vi "LatticeRamp_Generate_v4.vi"(5 "Input ramp":T4={"lattice ramp"=[{"dt"="0.010", "formula"="0.0"}, {"dt"="0.010", "formula"="f"}, {"dt"="0.010", "formula"="sin(2*pi*100*t)+1"}, {"dt"="0.010", "formula"="1-f"}], "Output"=[{"Time Values"=[0.0, 7.4775e-05, 0.004952823780487805, 0.009830872560975609, 0.014708921341463415, 0.01958697012195122, 0.024465018902439024, 0.02934306768292683, 0.034221116463414636, 0.03909916524390244, 0.04397721402439025, 0.04885526280487805, 0.05373331158536586, 0.05861136036585366, 0.06348940914634146, 0.06836745792682927, 0.07324550670731708, 0.07812355548780488, 0.08300160426829269, 0.0878796530487805, 0.09275770182926829, 0.0976357506097561, 0.10251379939024391, 0.10739184817073172, 0.11226989695121951, 0.11714794573170732, 0.12202599451219513, 0.12690404329268293, 0.13178209207317074, 0.13666014085365855, 0.14153818963414636, 0.14641623841463416, 0.15129428719512195, 0.15617233597560976, 0.16105038475609756, 0.16592843353658537, 0.17080648231707318, 0.175684531097561, 0.1805625798780488, 0.18544062865853658, 0.1903186774390244, 0.1951967262195122, 0.200074775, 0.20014955, 0.20504955, 0.20994955, 0.210024325, 0.710524325, 1.211024325, 1.2110991, 1.2111991, 1.2112991], [-2.42, -2.42, -2.274644675841946, -2.209161629253642, -2.1550360243297555, -2.1059224619056875, -2.059369043262097, -2.0141023350157363, -1.9693429960844966, -1.9245576980378343, -1.8793492014535609, -1.8334007369631589, -1.7864449866349144, -1.7382453890245562, -1.6885840896654052, -1.6372536703029252, -1.5840511006332372, -1.5287730108087192, -1.4712117270212386, -1.4111516989449542, -1.3483660486208333, -1.2826130206804396, -1.2136321308648308, -1.14113980114949, -1.064824236902151, -0.9843392409185628, -0.899296562073762, -0.809256226432418, -0.7137140678937928, -0.6120853153944805, -0.503682519181236, -0.38768515498282585, -0.26309663961745094, -0.1286816451362946, 0.017128703533097003, 0.17638664147159178, 0.35187774884695067, 0.547568099398879, 0.7694813778413232, 1.027657386702481, 1.3414861643128648, 1.7605557393789637, 2.8, 2.8, 2.8, 2.8, 2.8, 2.8, 2.8, -2.42, -2.42, -2.42]}, {"Time Values"=[0.0, 7.4775e-05, 0.004952823780487805, 0.009830872560975609, 0.014708921341463415, 0.01958697012195122, 0.024465018902439024, 0.02934306768292683, 0.034221116463414636, 0.03909916524390244, 0.04397721402439025, 0.04885526280487805, 0.05373331158536586, 0.05861136036585366, 0.06348940914634146, 0.06836745792682927, 0.07324550670731708, 0.07812355548780488, 0.08300160426829269, 0.0878796530487805, 0.09275770182926829, 0.0976357506097561, 0.10251379939024391, 0.10739184817073172, 0.11226989695121951, 0.11714794573170732, 0.12202599451219513, 0.12690404329268293, 0.13178209207317074, 0.13666014085365855, 0.14153818963414636, 0.14641623841463416, 0.15129428719512195, 0.15617233597560976, 0.16105038475609756, 0.16592843353658537, 0.17080648231707318, 0.175684531097561, 0.1805625798780488, 0.18544062865853658, 0.1903186774390244, 0.1951967262195122, 0.200074775, 0.20014955, 0.20504955, 0.20994955, 0.210024325, 0.710524325, 1.211024325, 1.2110991, 1.2111991, 1.2112991], [0.0, -0.0, 0.001911981360536598, 0.004019900016154734, 0.006343835359047381, 0.008905924490689818, 0.011730573093137419, 0.01484468791013227, 0.018277933052562964, 0.022063012569765436, 0.026235981978353178, 0.030836591716105637, 0.03590866579255229, 0.04150051924316252, 0.04766541836368316, 0.05446208810867599, 0.06195527148757928, 0.0702163462869304, 0.07932400499345772, 0.08936500439478239, 0.10043499199819844, 0.11263941713974554, 0.12609453546252153, 0.1409285163325908, 0.15728266374139496, 0.17531276232461152, 0.19519056131922613, 0.21710541059454333, 0.24126606434146913, 0.2679026696014608, 0.2972689585772668, 0.3296446656087423, 0.36533819183711563, 0.40468954294049037, 0.44807356792455355, 0.4959035298202305, 0.5486350423016632, 0.6067704097235386, 0.6708634119196445, 0.7415245793411871, 0.8194270087842359, 0.905312775105144, 1.0, 1.0, 1.0, 1.0, 1.0, 1.0, 1.0, 0.0, 0.0, 0.0]}], "SRS Selection"=enum."1550 Vertical"}, 6 "Current Variable settings":T1[](array[typedef])=[{"Procedure variable"="delay", "Value"=2.3}, {"Procedure variable"="z", "Value"=0.0}], 7 "error in (no error)":errorcluster) -> (0 "Output ramp":T4={"lattice ramp"=[{"dt"="0.010", "formula"="0.0"}, {"dt"="0.010", "formula"="f"}, {"dt"="0.010", "formula"="sin(2*pi*100*t)+1"}, {"dt"="0.010", "formula"="1-f"}], "Output"=[{"Time Values"=[0.0, 2.475e-06, 0.000771248076923077, 0.001540021153846154, 0.0023087942307692313, 0.003077567307692308, 0.003846340384615385, 0.0046151134615384625, 0.005383886538461539, 0.006152659615384616, 0.006921432692307693, 0.00769020576923077, 0.008458978846153847, 0.009227751923076925, 0.009996525000000001, 0.009999000000000001, 0.010768344230769231, 0.011537688461538463, 0.012307032692307693, 0.013076376923076925, 0.013845721153846155, 0.014615065384615385, 0.015384409615384616, 0.016153753846153848, 0.016923098076923077, 0.01769244230769231, 0.01846178653846154, 0.01923113076923077, 0.020000475, 0.02000295, 0.02018466, 0.020366369999999998, 0.02054808, 0.020729789999999998, 0.0209115, 0.021093209999999998, 0.02127492, 0.021456629999999997, 0.02163834, 0.02182005, 0.02200176, 0.022183469999999997, 0.02236518, 0.02254689, 0.022728599999999998, 0.02291031, 0.023092019999999998, 0.02327373, 0.023455439999999998, 0.02363715, 0.023818859999999997, 0.02400057, 0.02418228, 0.02436399, 0.0245457, 0.02472741, 0.02490912, 0.025090829999999998, 0.02527254, 0.025454249999999998, 0.02563596, 0.02581767, 0.02599938, 0.026181089999999997, 0.0263628, 0.02654451, 0.02672622, 0.02690793, 0.027089639999999998, 0.02727135, 0.02745306, 0.02763477, 0.027816479999999998, 0.02799819, 0.0281799, 0.02836161, 0.028543319999999997, 0.02872503, 0.02890674, 0.029088450000000002, 0.02927016, 0.029451869999999998, 0.02963358, 0.02981529, 0.029997, 0.029999474999999998, 0.03076881923076923, 0.03153816346153846, 0.03230750769230769, 0.03307685192307692, 0.03384619615384615, 0.03461554038461538, 0.03538488461538461, 0.036154228846153845, 0.03692357307692307, 0.03769291730769231, 0.03846226153846154, 0.039231605769230765, 0.04000094999999999], [0.0, 0.0, 0.0, 0.0, 0.0, 0.0, 0.0, 0.0, 0.0, 0.0, 0.0, 0.0, 0.0, 0.0, 0.0, 0.0, 0.07692307692307693, 0.15384615384615385, 0.23076923076923078, 0.3076923076923077, 0.38461538461538464, 0.46153846153846156, 0.5384615384615384, 0.6153846153846154, 0.6923076923076923, 0.7692307692307693, 0.8461538461538461, 0.9230769230769231, 1.0, 1.0, 1.1139238800498696, 1.226364353008397, 1.335857327283306, 1.4409770907726172, 1.5403548751151055, 1.6326966784741854, 1.716800114784089, 1.7915700700636759, 1.8560329619364289, 1.9093494166828902, 1.950825198757172, 1.9799202504538926, 1.9962557240197008, 1.9996189146440044, 1.9899660300962418, 1.9674227609461497, 1.9322826439421659, 1.8850032398584795, 1.8262001755791255, 1.7566391279973623, 1.6772258541082894, 1.588994397113228, 1.4930936221046294, 1.3907722566508556, 1.2833626310679325, 1.1722633300968168, 1.0589209818793124, 0.9448114213590806, 0.8314204733797951, 0.7202246057044277, 0.6126717038734424, 0.5101622182331631, 0.41403092861958235, 0.3255295641403312, 0.245810504363279, 0.17591177413920145, 0.11674352744147698, 0.06907619621725625, 0.03353045856433845, 0.010569156858512452, 0.0004912710657166697, 0.003428025712751026, 0.019341181207819358, 0.048023531759680216, 0.0891016034119837, 0.14204051706158627, 0.20615095313930343, 0.2805981272657321, 0.36441266000978945, 0.4565031992144406, 0.5556706305338442, 0.6606236911459755, 0.7699957833339905, 0.8823627690060711, 0.9962615134506403, 1.0, 0.9230769230769231, 0.8461538461538461, 0.7692307692307692, 0.6923076923076923, 0.6153846153846154, 0.5384615384615384, 0.46153846153846156, 0.3846153846153846, 0.3076923076923077, 0.23076923076923073, 0.15384615384615385, 0.07692307692307687, 0.0]}, {"Time Values"=[0.0, 2.475e-06, 0.000771248076923077, 0.001540021153846154, 0.0023087942307692313, 0.003077567307692308, 0.003846340384615385, 0.0046151134615384625, 0.005383886538461539, 0.006152659615384616, 0.006921432692307693, 0.00769020576923077, 0.008458978846153847, 0.009227751923076925, 0.009996525000000001, 0.009999000000000001, 0.010768344230769231, 0.011537688461538463, 0.012307032692307693, 0.013076376923076925, 0.013845721153846155, 0.014615065384615385, 0.015384409615384616, 0.016153753846153848, 0.016923098076923077, 0.01769244230769231, 0.01846178653846154, 0.01923113076923077, 0.020000475, 0.02000295, 0.02018466, 0.020366369999999998, 0.02054808, 0.020729789999999998, 0.0209115, 0.021093209999999998, 0.02127492, 0.021456629999999997, 0.02163834, 0.02182005, 0.02200176, 0.022183469999999997, 0.02236518, 0.02254689, 0.022728599999999998, 0.02291031, 0.023092019999999998, 0.02327373, 0.023455439999999998, 0.02363715, 0.023818859999999997, 0.02400057, 0.02418228, 0.02436399, 0.0245457, 0.02472741, 0.02490912, 0.025090829999999998, 0.02527254, 0.025454249999999998, 0.02563596, 0.02581767, 0.02599938, 0.026181089999999997, 0.0263628, 0.02654451, 0.02672622, 0.02690793, 0.027089639999999998, 0.02727135, 0.02745306, 0.02763477, 0.027816479999999998, 0.02799819, 0.0281799, 0.02836161, 0.028543319999999997, 0.02872503, 0.02890674, 0.029088450000000002, 0.02927016, 0.029451869999999998, 0.02963358, 0.02981529, 0.029997, 0.029999474999999998, 0.03076881923076923, 0.03153816346153846, 0.03230750769230769, 0.03307685192307692, 0.03384619615384615, 0.03461554038461538, 0.03538488461538461, 0.036154228846153845, 0.03692357307692307, 0.03769291730769231, 0.03846226153846154, 0.039231605769230765, 0.04000094999999999], [0.0, 0.0, 0.0, 0.0, 0.0, 0.0, 0.0, 0.0, 0.0, 0.0, 0.0, 0.0, 0.0, 0.0, 0.0, 0.0, 0.07692307692307693, 0.15384615384615385, 0.23076923076923078, 0.3076923076923077, 0.38461538461538464, 0.46153846153846156, 0.5384615384615384, 0.6153846153846154, 0.6923076923076923, 0.7692307692307693, 0.8461538461538461, 0.9230769230769231, 1.0, 1.0, 1.1139238800498696, 1.226364353008397, 1.335857327283306, 1.4409770907726172, 1.5403548751151055, 1.6326966784741854, 1.716800114784089, 1.7915700700636759, 1.8560329619364289, 1.9093494166828902, 1.950825198757172, 1.9799202504538926, 1.9962557240197008, 1.9996189146440044, 1.9899660300962418, 1.9674227609461497, 1.9322826439421659, 1.8850032398584795, 1.8262001755791255, 1.7566391279973623, 1.6772258541082894, 1.588994397113228, 1.4930936221046294, 1.3907722566508556, 1.2833626310679325, 1.1722633300968168, 1.0589209818793124, 0.9448114213590806, 0.8314204733797951, 0.7202246057044277, 0.6126717038734424, 0.5101622182331631, 0.41403092861958235, 0.3255295641403312, 0.245810504363279, 0.17591177413920145, 0.11674352744147698, 0.06907619621725625, 0.03353045856433845, 0.010569156858512452, 0.0004912710657166697, 0.003428025712751026, 0.019341181207819358, 0.048023531759680216, 0.0891016034119837, 0.14204051706158627, 0.20615095313930343, 0.2805981272657321, 0.36441266000978945, 0.4565031992144406, 0.5556706305338442, 0.6606236911459755, 0.7699957833339905, 0.8823627690060711, 0.9962615134506403, 1.0, 0.9230769230769231, 0.8461538461538461, 0.7692307692307692, 0.6923076923076923, 0.6153846153846154, 0.5384615384615384, 0.46153846153846156, 0.3846153846153846, 0.3076923076923077, 0.23076923076923073, 0.15384615384615385, 0.07692307692307687, 0.0]}], "SRS Selection"=enum."1550 Vertical"}, 1 "Output time":dbl[](array[numeric])=[0.0, 2.475e-06, 0.000771248076923077, 0.001540021153846154, 0.0023087942307692313, 0.003077567307692308, 0.003846340384615385, 0.0046151134615384625, 0.005383886538461539, 0.006152659615384616, 0.006921432692307693, 0.00769020576923077, 0.008458978846153847, 0.009227751923076925, 0.009996525000000001, 0.009999000000000001, 0.010768344230769231, 0.011537688461538463, 0.012307032692307693, 0.013076376923076925, 0.013845721153846155, 0.014615065384615385, 0.015384409615384616, 0.016153753846153848, 0.016923098076923077, 0.01769244230769231, 0.01846178653846154, 0.01923113076923077, 0.020000475, 0.02000295, 0.02018466, 0.020366369999999998, 0.02054808, 0.020729789999999998, 0.0209115, 0.021093209999999998, 0.02127492, 0.021456629999999997, 0.02163834, 0.02182005, 0.02200176, 0.022183469999999997, 0.02236518, 0.02254689, 0.022728599999999998, 0.02291031, 0.023092019999999998, 0.02327373, 0.023455439999999998, 0.02363715, 0.023818859999999997, 0.02400057, 0.02418228, 0.02436399, 0.0245457, 0.02472741, 0.02490912, 0.025090829999999998, 0.02527254, 0.025454249999999998, 0.02563596, 0.02581767, 0.02599938, 0.026181089999999997, 0.0263628, 0.02654451, 0.02672622, 0.02690793, 0.027089639999999998, 0.02727135, 0.02745306, 0.02763477, 0.027816479999999998, 0.02799819, 0.0281799, 0.02836161, 0.028543319999999997, 0.02872503, 0.02890674, 0.029088450000000002, 0.02927016, 0.029451869999999998, 0.02963358, 0.02981529, 0.029997, 0.029999474999999998, 0.03076881923076923, 0.03153816346153846, 0.03230750769230769, 0.03307685192307692, 0.03384619615384615, 0.03461554038461538, 0.03538488461538461, 0.036154228846153845, 0.03692357307692307, 0.03769291730769231, 0.03846226153846154, 0.039231605769230765, 0.04000094999999999] format="%#_6p", 2 "Output calculated":dbl[](array[numeric])=[0.0, 0.0, 0.0, 0.0, 0.0, 0.0, 0.0, 0.0, 0.0, 0.0, 0.0, 0.0, 0.0, 0.0, 0.0, 0.0, 0.07692307692307693, 0.15384615384615385, 0.23076923076923078, 0.3076923076923077, 0.38461538461538464, 0.46153846153846156, 0.5384615384615384, 0.6153846153846154, 0.6923076923076923, 0.7692307692307693, 0.8461538461538461, 0.9230769230769231, 1.0, 1.0, 1.1139238800498696, 1.226364353008397, 1.335857327283306, 1.4409770907726172, 1.5403548751151055, 1.6326966784741854, 1.716800114784089, 1.7915700700636759, 1.8560329619364289, 1.9093494166828902, 1.950825198757172, 1.9799202504538926, 1.9962557240197008, 1.9996189146440044, 1.9899660300962418, 1.9674227609461497, 1.9322826439421659, 1.8850032398584795, 1.8262001755791255, 1.7566391279973623, 1.6772258541082894, 1.588994397113228, 1.4930936221046294, 1.3907722566508556, 1.2833626310679325, 1.1722633300968168, 1.0589209818793124, 0.9448114213590806, 0.8314204733797951, 0.7202246057044277, 0.6126717038734424, 0.5101622182331631, 0.41403092861958235, 0.3255295641403312, 0.245810504363279, 0.17591177413920145, 0.11674352744147698, 0.06907619621725625, 0.03353045856433845, 0.010569156858512452, 0.0004912710657166697, 0.003428025712751026, 0.019341181207819358, 0.048023531759680216, 0.0891016034119837, 0.14204051706158627, 0.20615095313930343, 0.2805981272657321, 0.36441266000978945, 0.4565031992144406, 0.5556706305338442, 0.6606236911459755, 0.7699957833339905, 0.8823627690060711, 0.9962615134506403, 1.0, 0.9230769230769231, 0.8461538461538461, 0.7692307692307692, 0.6923076923076923, 0.6153846153846154, 0.5384615384615384, 0.46153846153846156, 0.3846153846153846, 0.3076923076923077, 0.23076923076923073, 0.15384615384615385, 0.07692307692307687, 0.0], 3 "Delta t":dbl=2.475e-06 format="%_5e", 4 "error out":errorcluster)   [LabVIEW 2013, in "SubVIs.lvlib"]
uses:
  no caller/SubVIs.lvlib
  codes/DeviceVIs/SRSDevices.ctt
  codes/Controls.llb/Controls.lvlib
  codes/DeviceVIs/SRSRampControl_v4.ctl
  codes/TypeDefs/Active procedure variables.ctl
panel:
  out "Times":dbl[](array[numeric])=[0.00999405, 0.010001475, 0.00999405, 0.010001475]
  out "Computed steps":dbl=16158.0
  out "Assembeled steps":dbl=16161.999999999996 format="%#_7f"
  out "Requested time":dbl=0.04 format="%#_7e"
  out "Segments":dbl=98.0
  out "Steps":dbl=16161.616161616163
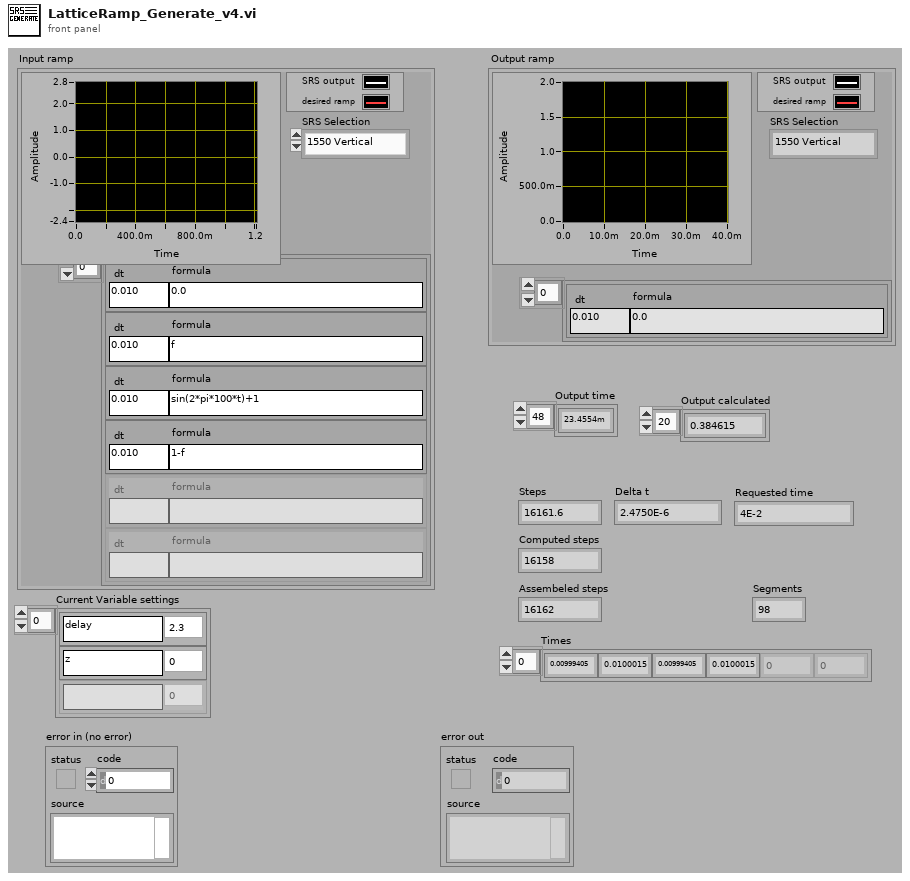
[diagram p1: front panel]
types:
  T1 = typedef "Active procedure variables.ctl" = cluster{"Procedure variable":string, "Value":dbl}
  T2 = typedef "Controls.lvlib/SRSRampControl_v4.ctl" = cluster{"dt":string, "formula":string}
  T3 = typedef "Controls.lvlib/SRSDevices.ctt" = enum16{"1550 Vertical", "Bragg Agilent", "Bragg PTS", "Acc. Intensity"}
  T4 = cluster{"lattice ramp":T2[], "Output":cluster{"Time Values":dbl[], dbl[]}[], "SRS Selection":T3}
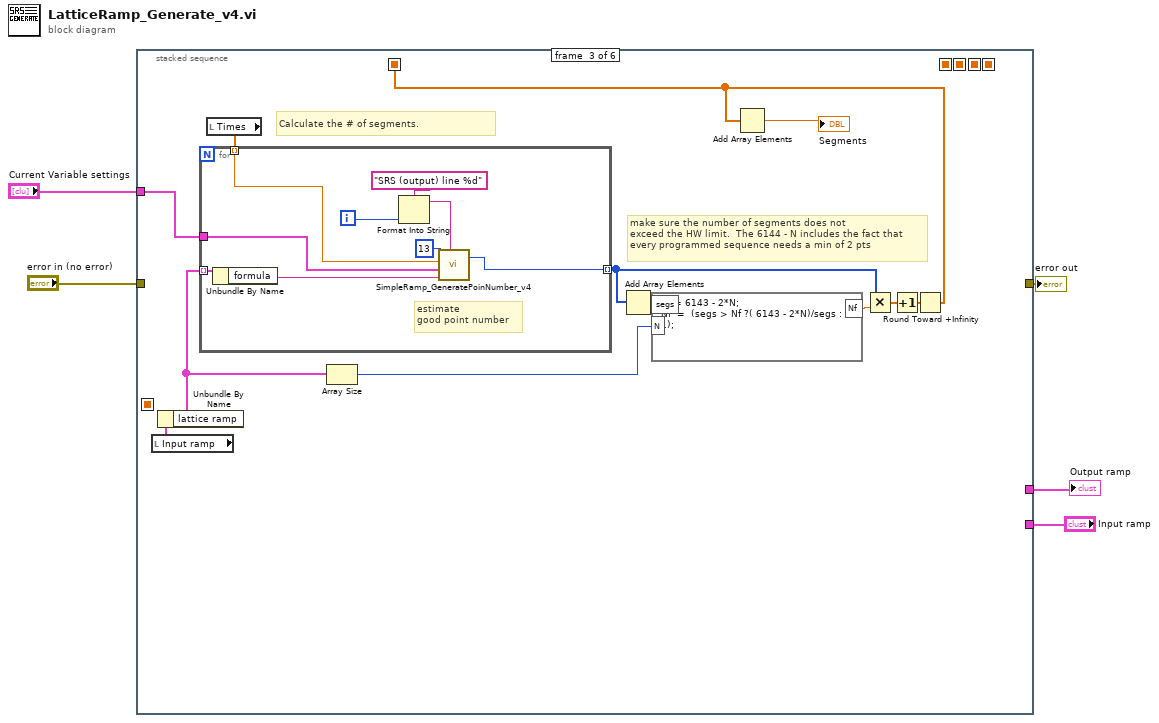
[diagram p0: block diagram]
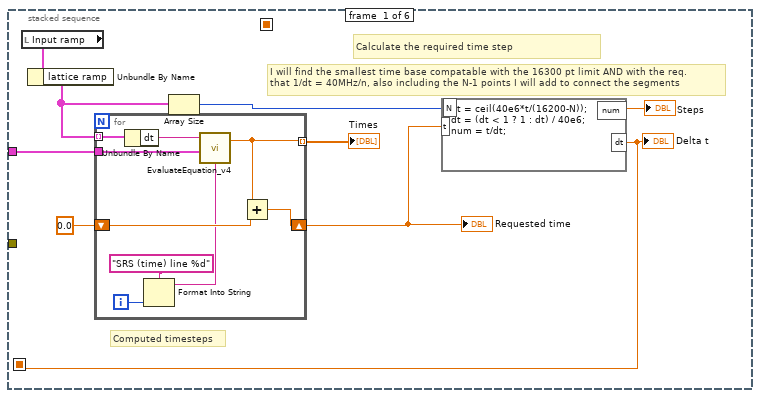
[diagram p2: hidden frame]
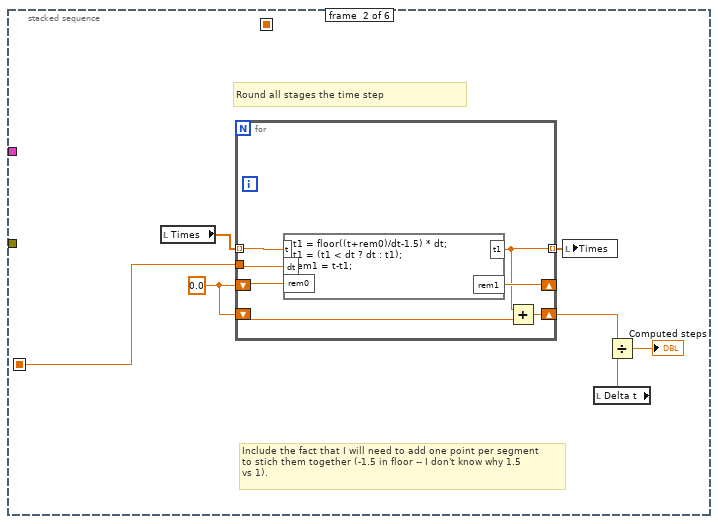
[diagram p3: hidden frame]
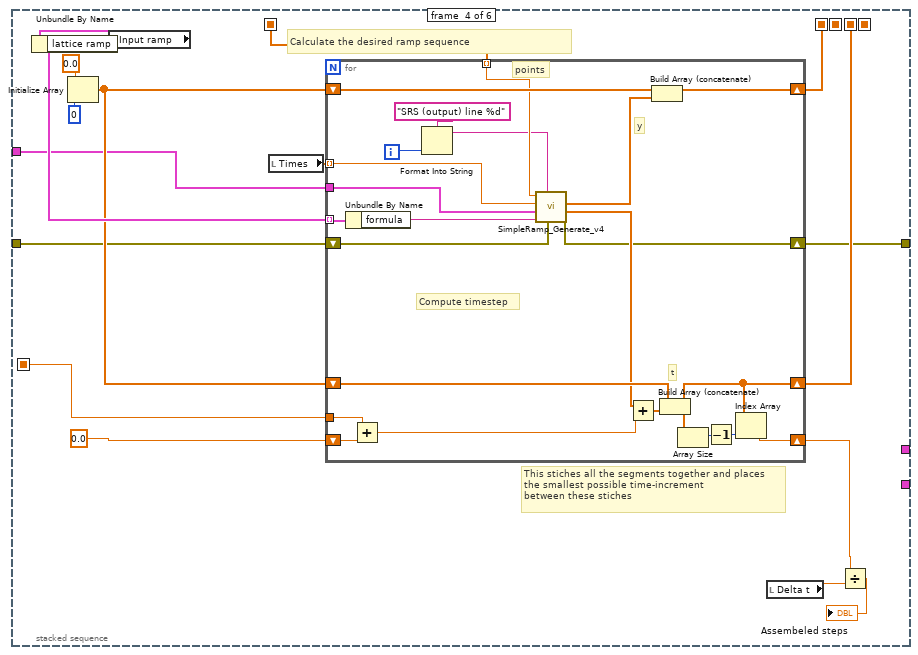
[diagram p4: hidden frame]
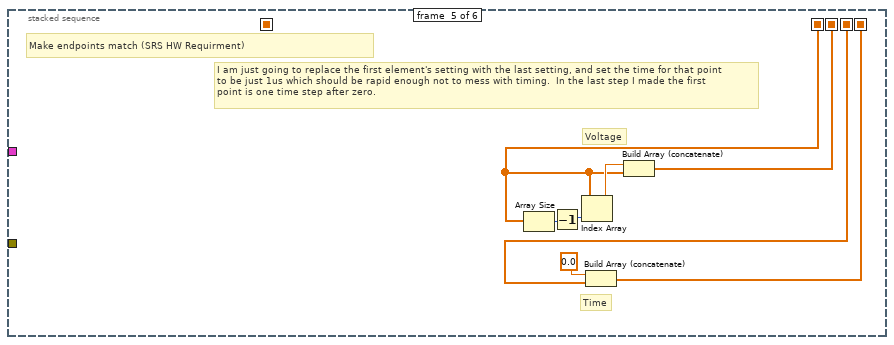
[diagram p5: hidden frame]
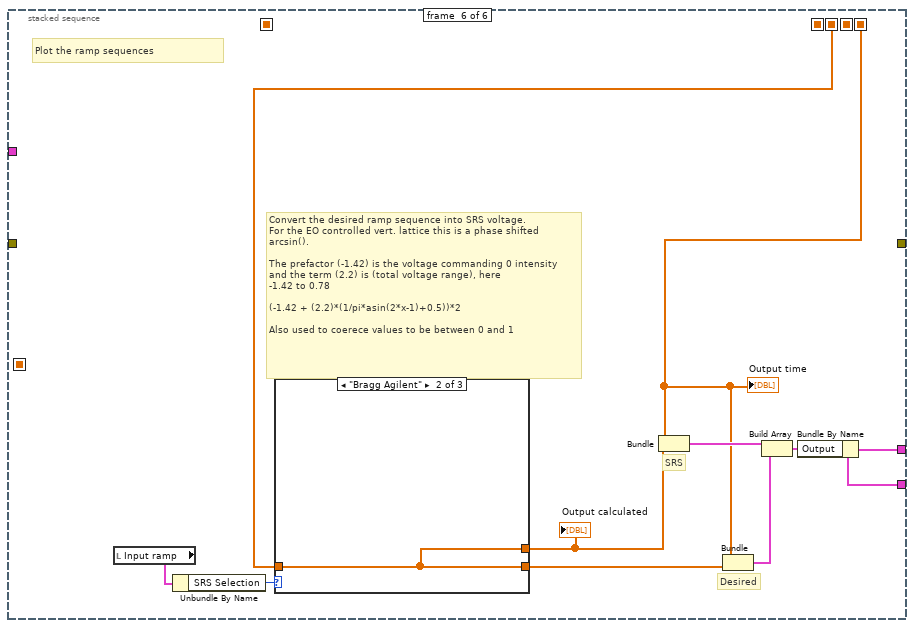
[diagram p6: hidden frame]
diagram:
  n1 = stacked-sequence {
    seq-local: [_ _ _ w71 _ _] -> [_ _ _ _ w102 _]
    seq-local: [_ _ _ w64 _ _] -> [_ _ _ _ w101 _]
    seq-local: [w9 _ _ _ _ _] -> [_ w30 _ w69 _ _]
    seq-local: [_ _ w42 _ _ _] -> [_ _ _ w68 _ _]
    seq-local: [_ _ _ _ w100 _] -> [_ _ _ _ _ w111]
    seq-local: [_ _ _ _ w99 _] -> [_ _ _ _ _ w109]
    tunnel: [_ _ _ _ _ w114] -> w5
    tunnel: "Input ramp" -> [_ _ _ _ _ w107]
    tunnel: "Current Variable settings" -> [w7 _ w39 w62 _ _]
    tunnel: "error in (no error)" -> [_ _ _ w61 _ _]
    tunnel: [_ _ _ w60 _ _] -> w1
    frame #0 {
      # "Computed timesteps"
      # "I will find the smallest time base compatable with the 16300 pt limit AND with the req. \nthat 1/dt = 40MHz/n, also including the N-1 points I will add to connect the segments"
      # "Calculate the required time step"
      n2 = local read "Input ramp"() -> (w8:T4)
      n3 = Unbundle By Name(w8) -> ("lattice ramp"=w11:T2[])
      n4 = for {
        tunnel: w11 -> [w23] mode=indexing
        shift-right: [w21] -> w10
        shift-left: 0.0 -> [w22]
        tunnel: w7 -> [w19]
        tunnel: [w18] -> w6 mode=indexing
        i -> [w16]
        n5 = Unbundle By Name(w23) -> ("dt"=w20:string)
        n6 = Format Into String(format string="SRS (time) line %d", w16) -> (resulting string=w15:string)  [unwired: 2 in, 1 out]
        n7 = call "EvaluateEquation_v4.vi"("Error Locator"=w15, "Current Variable settings"=w19, "formula"=w20) -> ("y value"=w18:dbl)  [unwired: 1 in, 1 out]
        n8 = Add(x=w18, y=w22) -> (x+y=w21:dbl)
      }
      "Requested time" <- w10
      "Times" <- w6
      n9 = Array Size(array=w11) -> (size(s)=w13:i32)
      n10 = formula code="dt = ceil(40e6*t/(16200-N));\ndt = (dt < 1 ? 1 : dt) / 40e6;\nnum = t/dt;"("t"=w10, "N"=w13) -> ("dt"=w9:dbl, "num"=→"Steps":dbl)
      "Delta t" <- w9
    }
    frame #1 {
      w29 = 0.0
      # "Include the fact that I will need to add one point per segment\nto stich them together (-1.5 in floor -- I don't know why 1.5\nvs 1)."
      # "Round all stages the time step"
      n11 = local read "Times"() -> (w25:dbl[])
      n12 = for {
        shift-right: [w37] -> _
        shift-left: w29 -> [w36]
        tunnel: w30 -> [w35]
        shift-right: [w33] -> w27
        shift-left: w29 -> [w34]
        tunnel: w25 -> [w32] mode=indexing
        tunnel: [w31] -> w24 mode=indexing
        n13 = formula code="t1 = floor((t+rem0)/dt-1.5) * dt;\nt1 = (t1 < dt ? dt : t1);\nrem1 = t-t1;"("t"=w32, "dt"=w35, "rem0"=w36) -> ("t1"=w31:dbl, "rem1"=w37:dbl)
        n14 = Add(x=w31, y=w34) -> (x+y=w33:dbl)
      }
      n15 = local write "Times"(w24) -> ()
      n16 = local read "Delta t"() -> (w28:dbl)
      n17 = Divide(x=w27, y=w28) -> (x/y=→"Computed steps":dbl)
    }
    frame #2 {
      # "make sure the number of segments does not\nexceed the HW limit.  The 6144 - N includes the fact that\nevery programmed sequence needs a min of 2 pts"
      # "Calculate the # of segments."
      n18 = local read "Input ramp"() -> (w40:T4)
      n19 = Unbundle By Name(w40) -> ("lattice ramp"=w49:T2[])
      n20 = local read "Times"() -> (w38:dbl[])
      n21 = for {
        tunnel: w49 -> [w58] mode=indexing
        tunnel: [w56] -> w45 mode=indexing
        tunnel: w39 -> [w54]
        tunnel: w38 -> [w53] mode=indexing
        i -> [w51]
        # "estimate\ngood point number"
        n22 = Unbundle By Name(w58) -> ("formula"=w55:string)
        n23 = Format Into String(format string="SRS (output) line %d", w51) -> (resulting string=w50:string)  [unwired: 2 in, 1 out]
        n24 = call "SimpleRamp_GeneratePoinNumber_v4.vi"("Error Locator"=w50, "formula"=w55, "Current Variable settings"=w54, "dt"=w53, "Points"=13) -> ("Suggested point number"=w56:u32)  [unwired: 1 in, 1 out]
      }
      n25 = Array Size(array=w49) -> (size(s)=w44:i32)
      n26 = Add Array Elements(numeric array=w45) -> (sum=w48:u32)
      n27 = formula code="Nf = 6143 - 2*N;\nNf  =  (segs > Nf ?( 6143 - 2*N)/segs : 1);"("segs"=w48, "N"=w44) -> ("Nf"=w46:dbl)
      n28 = Multiply(x=w45, y=w46) -> (x*y=w47:dbl[])
      n29 = Increment(x=w47) -> (x+1=w43:dbl[])
      n30 = Round Toward +Infinity(x=w43) -> (ceil(x): smallest int >= x=w42:dbl[])
      n31 = Add Array Elements(numeric array=w42) -> (sum=→"Segments":dbl)
    }
    frame #3 {
      # "This stiches all the segments together and places \nthe smallest possible time-increment\nbetween these stiches"
      # "Calculate the desired ramp sequence"
      n32 = Initialize Array(0.0, 0) -> (w72:dbl[])
      n33 = local read "Input ramp"() -> (w63:T4)
      n34 = Unbundle By Name(w63) -> ("lattice ramp"=w75:T2[])
      n35 = local read "Times"() -> (w59:dbl[])
      n36 = for {
        tunnel: w75 -> [w87] mode=indexing
        shift-right: [w96] -> w71
        shift-left: w72 -> [w95]
        shift-right: [w92] -> w64
        shift-left: w72 -> [w97]
        shift-right: [w88] -> w65
        shift-left: 0.0 -> [w91]
        tunnel: w69 -> [w90]
        tunnel: w68 -> [w86] mode=indexing
        tunnel: w62 -> [w82]
        shift-right: [w83] -> w60
        shift-left: w61 -> [w80]
        tunnel: w59 -> [w79] mode=indexing
        i -> [w77]
        # "Compute timestep"
        # "points"
        # "t"
        # "y"
        n37 = Unbundle By Name(w87) -> ("formula"=w81:string)
        n38 = Add(x=w90, y=w91) -> (x+y=w89:dbl)
        n39 = Format Into String(format string="SRS (output) line %d", w77) -> (resulting string=w76:string)  [unwired: 2 in, 1 out]
        n40 = call "SimpleRamp_Generate_v4.vi"("error in (no error)"=w80, "Error Locator"=w76, "formula"=w81, "Current Variable settings"=w82, "dt"=w79, "Points"=w86) -> ("error out"=w83:errorcluster, "x values"=w84:dbl[], "y values"=w85:dbl[])  [unwired: 1 out]
        n41 = Add(x=w84, y=w89) -> (x+y=w98:dbl[])
        n42 = Build Array (concatenate)(w95, w85) -> (w96:dbl[])
        n43 = Build Array (concatenate)(w97, w98) -> (w92:dbl[])
        n44 = Array Size(array=w92) -> (size(s)=w94:i32)
        n45 = Decrement(x=w94) -> (x-1=w93:i32)
        n46 = Index Array(array=w92, index=w93) -> (element=w88:dbl)
      }
      n47 = local read "Delta t"() -> (w67:dbl)
      n48 = Divide(x=w65, y=w67) -> (x/y=→"Assembeled steps":dbl)
    }
    frame #4 {
      # "Time"
      # "Voltage"
      # "I am just going to replace the first element's setting with the last setting, and set the time for that point\nto be just 1us which should be rapid enough not to mess with timing.  In the last step I made the first\npoint is one time step after zero."
      # "Make endpoints match (SRS HW Requirment)"
      n49 = Array Size(array=w102) -> (size(s)=w106:i32)
      n50 = Decrement(x=w106) -> (x-1=w105:i32)
      n51 = Index Array(array=w102, index=w105) -> (element=w104:dbl)
      n52 = Build Array (concatenate)(0.0, w101) -> (w99:dbl[])
      n53 = Build Array (concatenate)(w104, w102) -> (w100:dbl[])
    }
    frame #5 {
      # "SRS"
      # "Desired"
      # "Plot the ramp sequences"
      # "Convert the desired ramp sequence into SRS voltage.\nFor the EO controlled vert. lattice this is a phase shifted\narcsin().\n\nThe prefactor (-1.42) is the voltage commanding 0 intensity\nand the term (2.2) is (total voltage range), here\n-1.42 to 0.78 \n\n(-1.42 +\t(2.2)*(1/pi*asin(2*x-1)+0.5))*2\n\nAlso used to coerece values to be between 0 and 1"
      n54 = local read "Input ramp"() -> (w108:T4)
      n55 = Unbundle By Name(w108) -> ("SRS Selection"=w113:T3)
      n56 = case shown="\"Bragg Agilent\"" w113 {
        tunnel: [w118 w119 w120] -> w112
        tunnel: [w118 w119 w120] -> w110
        tunnel: w111 -> [w118 w119 w120]
        frame "1550 Vertical", Default {
        }
        frame "Bragg Agilent" {
        }
        frame "Bragg PTS" {
        }
      }
      "Output calculated" <- w110
      n57 = Bundle(w109, w110) -> (w117:cluster{dbl[], dbl[]})  [unwired: 1 out]
      n58 = Bundle(w109, w112) -> (w116:cluster{dbl[], dbl[]})  [unwired: 1 out]
      n59 = Build Array(w117, w116) -> (w115:cluster{dbl[], dbl[]}[])
      n60 = Bundle By Name(cluster=w107, "Output"=w115) -> (w114:T4)
      "Output time" <- w109
    }
  }
  "Output ramp" <- w5
  "error out" <- w1
